vi "Player Info.vi"(11 "Snail In":refnum<class "Random Location.lvclass">) -> (1 "Victory Speech":string, 2 "Name":string, 3 "Snail Out":refnum<class "Random Location.lvclass">)   [LabVIEW 2015, in "Random Location.lvclass"]
uses:
  Random Location.lvclass
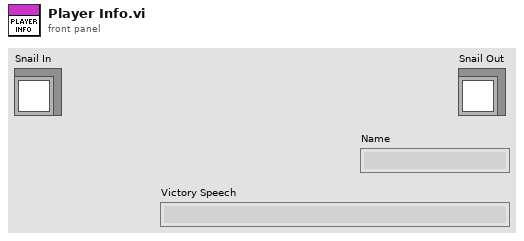
[diagram p1: front panel]
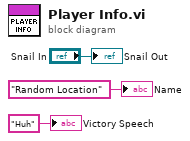
[diagram p0: block diagram]
diagram:
  "Snail Out" <- "Snail In"
  "Name" <- "Random Location" ("Name")
  "Victory Speech" <- "Huh" ("Victory Speech")
